vi "Excel_Set_Cell_Format.vi"(8 "error in (no error)":errorcluster, 9 "Bookmark/NamedCell":string, 10 "number format":string, 11 "report in":refnum<class "NI_report.lvclass">) -> (0 "error out":errorcluster, 3 "report out":refnum<class "NI_report.lvclass">)   [LabVIEW 2010, in "NI_ReportGenerationToolkit.lvlib"]
uses:
  <vilib>/addons/_office/NI_ReportGenerationToolkit.lvlib
  <vilib>/Utility/NIReport.llb/NI_report.lvclass
  <vilib>/Utility/NIReport.llb/Excel/NI_Excel.lvclass
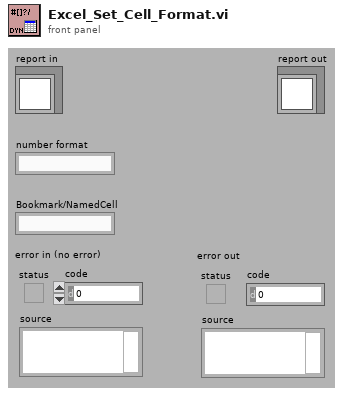
[diagram p1: front panel]
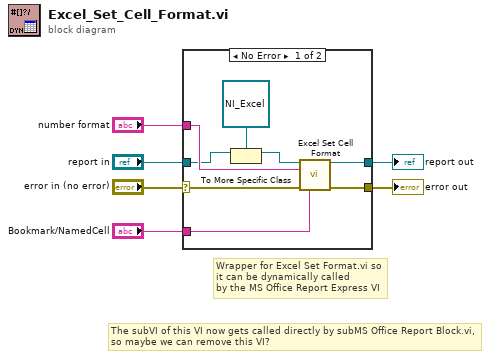
[diagram p0: block diagram]
diagram:
  # "The subVI of this VI now gets called directly by subMS Office Report Block.vi,\nso maybe we can remove this VI?"
  # "Wrapper for Excel Set Format.vi so\nit can be dynamically called\nby the MS Office Report Express VI"
  n1 = case shown="No Error" "error in (no error)" {
    selector: "error in (no error)" -> [w10 w15]
    tunnel: [w14 w16] -> w6
    tunnel: "report in" -> [w8 w16]
    tunnel: "number format" -> [w13 _]
    tunnel: "Bookmark/NamedCell" -> [w12 _]
    tunnel: [w11 w15] -> w2
    frame No Error {
      n2 = To More Specific Class(target class=refnum<class "NI_Excel.lvclass"> refnum ("report in"), reference=w8) -> (specific class reference=w7:refnum<class "NI_Excel.lvclass">)  [unwired: 1 in, 1 out]
      n3 = call <vilib>:"Excel Set Cell Format.vi"("report in"=w7, "number format"=w13, "error in (no error)"=w10, "name (\"\")"=w12) -> ("report out"=w14:refnum<class "NI_report.lvclass">, "error out"=w11:errorcluster)  [unwired: 10 in]
    }
    frame Error {
    }
  }
  "report out" <- w6
  "error out" <- w2
